vi "RemoveAllParentheses.vi"(1 "Script in":string) -> (0 "Script out":string)   [LabVIEW 2012]
panel:
  out "Array":string[](array[string])
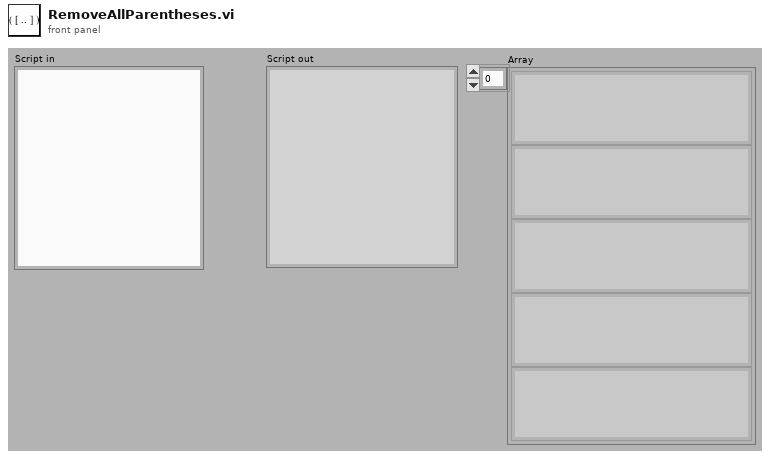
[diagram p1: front panel]
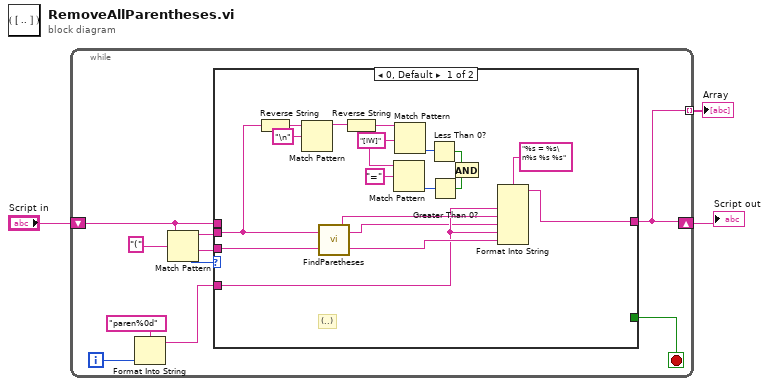
[diagram p0: block diagram]
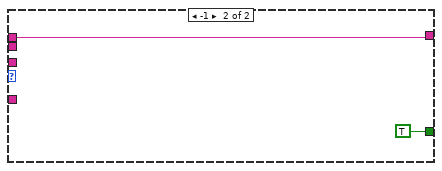
[diagram p2: hidden frame]
diagram:
  n1 = while {
    shift-right: [w5] -> w2
    shift-left: "Script in" -> [w6]
    tunnel: [w5] -> w1 mode=indexing
    i -> [w9]
    stop <- w7 stop-if-true
    n2 = Format Into String(format string="paren%0d" ("Script"), w9) -> (resulting string=w8:string)  [unwired: 2 in, 1 out]
    n3 = Match Pattern(string=w6, regular expression="(") -> (before substring=w11:string, after substring=w12:string, offset past match=w4:i32)  [unwired: 1 in, 1 out]
    n4 = case shown="0, Default" w4 {
      tunnel: [w26 w31] -> w5
      tunnel: w8 -> [w27 _]
      tunnel: w11 -> [w25 _]
      tunnel: w12 -> [w30 _]
      tunnel: [_ TRUE] -> w7
      tunnel: w6 -> [_ w31]
      frame 0, Default {
        # "(..)"
        n5 = Reverse String(1:w25) -> (0:w24:string)
        n6 = Match Pattern(string=w24, regular expression="\n") -> (before substring=w22:string)  [unwired: 1 in, 3 out]
        n7 = call <userlib>:"FindParetheses.vi"("String in"=w30) -> ("rest"=w29:string, "parentetical"=w28:string)
        n8 = Reverse String(1:w22) -> (0:w19:string)
        n9 = Match Pattern(string=w19, regular expression="=") -> (offset past match=w17:i32)  [unwired: 1 in, 3 out]
        n10 = Match Pattern(string=w19, regular expression="[IW]") -> (offset past match=w21:i32)  [unwired: 1 in, 3 out]
        n11 = Less Than 0?(x=w21) -> (x < 0?=w16:bool)
        n12 = Greater Than 0?(x=w17) -> (x > 0?=w15:bool)
        n13 = And(x=w16, y=w15) -> ()  [unwired: 1 out]
        n14 = Format Into String(format string="%s = %s\n%s %s %s", w27, w28, w25, w27, w29) -> (resulting string=w26:string)  [unwired: 2 in, 1 out]
      }
      frame -1 {
      }
    }
  }
  "Script out" <- w2
  "Array" <- w1
